vi "update DO.vi"(11 "Control":u8) -> ()   [LabVIEW 2015]
uses:
  <vilib>/rvi/eio/common/nirviEmuTemplateMethod_errors.vi
  <vilib>/eio/EIONode/EIONode.xnode
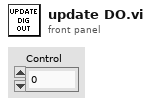
[diagram p1: front panel]
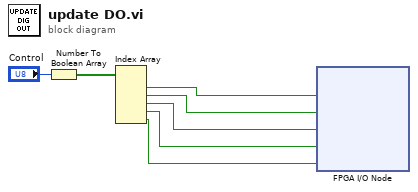
[diagram p0: block diagram]
diagram:
  n1 = Number To Boolean Array(number="Control") -> (Boolean array=w6:bool[])
  n2 = Index Array(array=w6) -> (element #1=w5:bool, element #2=w4:bool, element #3=w3:bool, element #4=w2:bool, element #5=w1:bool)  [unwired: 5 in]
  n3 = xnode "FPGA I/O Node"("PXI_Trig2"=w5, "PXI_Trig3"=w4, "PXI_Trig4"=w3, "PXI_Trig5"=w2, "PXI_Trig6"=w1) -> ()  [unwired: 5 in, 5 out]
